vi "Open.vi"(8 "error in (no error)":errorcluster, 10 "Update Rate (4Hz-100Hz)":u8=100, 11 "navX - Interface in":refnum<class "navX - Interface.lvclass">) -> (0 "error out":errorcluster, 3 "navX - Interface out":refnum<class "navX - Interface.lvclass">)   [LabVIEW 2015, in "navX Library v3.lvlib" / "navX - Interface.lvclass"]
uses:
  navX - Interface.lvclass
  navX Registry Cache/navX Registry Cache.lvclass
  _TypeDefs/NotificationPacketTypeDef.ctl
  _TypeDefs/NotificationActionsTypeDef.ctl
  navX - Interface.lvclass/navX - Interface.ctl
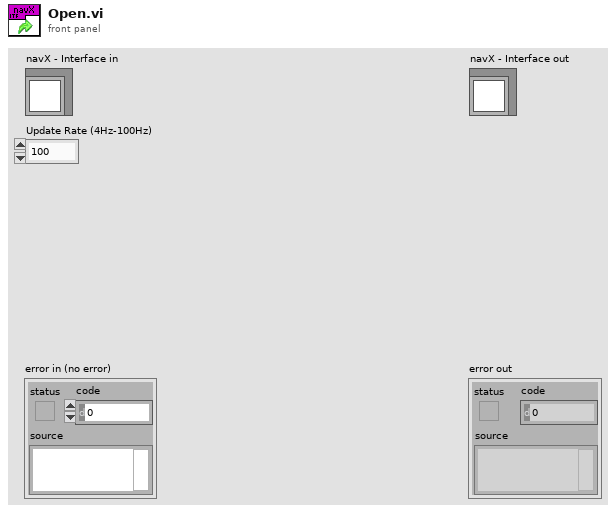
[diagram p1: front panel]
types:
  T1 = typedef "navX Library v3.lvlib/navX - Interface.lvclass/NotificationPacketTypeDef.ctl" = cluster{"Notification Action":T2, "Notification Data":variant}
  T2 = typedef "navX Library v3.lvlib/navX - Interface.lvclass/NotificationActionsTypeDef.ctl" = enum16{"UNKNOWN", "Stop Processing Loop", "Reconfigure", "Zero"}
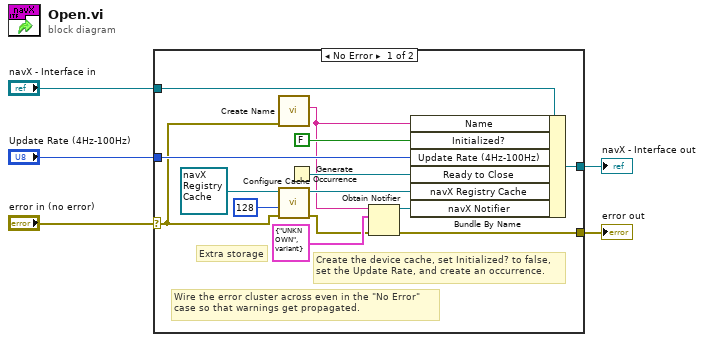
[diagram p0: block diagram]
diagram:
  n1 = case shown="No Error" "error in (no error)" {
    selector: "error in (no error)" -> [w7 w21]
    tunnel: [w9 w21] -> w4
    tunnel: [w14 w20] -> w2
    tunnel: "navX - Interface in" -> [w15 w20]
    tunnel: "Update Rate (4Hz-100Hz)" -> [w13 _]
    frame No Error {
      # "Extra storage"
      # "Create the device cache, set Initialized? to false,\nset the Update Rate, and create an occurrence."
      # "Wire the error cluster across even in the \"No Error\"\ncase so that warnings get propagated."
      n2 = call "Create Name.vi"("error in (no error)"=w7) -> ("Name"=w6:string)  [unwired: 9 in, 1 out]
      n3 = call "Configure Cache.vi"("error in (no error)"=w7, "Cache Size"=128 ("dimension size"), "navX Registry Cache in"=refnum<class "navX Registry Cache.lvclass"> refnum ("navX Library v3.lvlib:navX Registry Cache.lvclass")) -> ("error out"=w10:errorcluster, "navX Registry Cache out"=w18:refnum<class "navX Registry Cache.lvclass">)  [unwired: 7 in]
      n4 = Generate Occurrence() -> (w19:refnum<k4>)
      n5 = Obtain Notifier(name (unnamed)=w6, notification data type=T1 {"Notification Action"=enum."UNKNOWN", "Notification Data"=variant} ("Notification Packet"), error in (no error)=w10) -> (notifier out=w11:refnum<notifier>, error out=w9:errorcluster)  [unwired: 1 in, 1 out]
      n6 = Bundle By Name(cluster=w15, "Name"=w6, "Initialized?"=FALSE, "Update Rate (4Hz-100Hz)"=w13, "Ready to Close"=w19, "navX Registry Cache"=w18, "navX Notifier"=w11) -> (w14:refnum<class "navX - Interface.lvclass">)
    }
    frame Error {
    }
  }
  "error out" <- w4
  "navX - Interface out" <- w2
